vi "SECoP-doneLibrary.vi"(8 "error in (no error)":errorcluster, 11 "DLL path (in)":T1) -> (0 "error out":errorcluster, 3 "DLL path (out)":T1)   [LabVIEW 2023, in "SECoP.lvlib"]
doc: "<b>\"SECoP-doneLibrary.vi\"</b> should be called from \"SECoP-Exit.vi\" only.\n\n<b>DLL path</b> input and output of cluster from \"SECoP-Initialize.vi\""
uses:
  SECoP.lvlib
  Public/SECoP-libraries.ctl
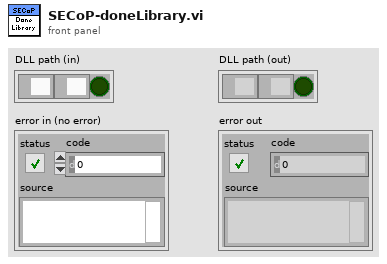
[diagram p1: front panel]
types:
  T1 = typedef "SECoP.lvlib/SECoP-libraries.ctl" = cluster{"serverDLL":path, "variantDLL":path, "cleanup_mode":bool}
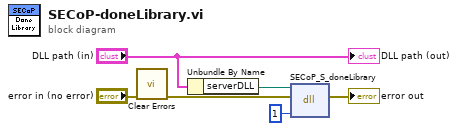
[diagram p0: block diagram]
diagram:
  n1 = call <vilib>:"Clear Errors.vi"("error in (no error)"="error in (no error)") -> ("error out"=w4:errorcluster)  [unwired: 5 in, 1 out]
  n2 = Unbundle By Name("DLL path (in)") -> ("serverDLL"=w1:path)
  n3 = dll-call lib="C:/Users/user/Desktop/x86_64/SECoP64.dll" fn="SECoP_S_doneLibrary"(path in=w1, error in=w4, "bNodesOnly"=1) -> (error out=→"error out":errorcluster)  [unwired: 3 in, 1 out]
  "DLL path (out)" <- "DLL path (in)"
